vi "Smart_Record_MTIF.vi"() -> ()   [LabVIEW 2019]
uses:
  <vilib>/vision/driver/IMAQdx.llb/IMAQdx Acquisition Mode.ctl
  <vilib>/vision/driver/IMAQdx.llb/IMAQdx Buffer Number Mode.ctl
  <vilib>/vision/driver/NI_Vision_Acquisition_Software.lvlib
  <resource>/objmgr/imaqdx.rc
  <vilib>/vision/NI_Vision_Development_Module.lvlib
panel:
  out "Data Valid":bool
  in  "Centroid Distance Threshold":sgl=5.0
  in  "Initial SD Threshold":sgl=4.0
  in  "SD Threshold Ratio for Stop":sgl=1.2
  in  "SD Threshold Ratio for Start":sgl=1.5
  out "Writing":bool
  in  "Number of Buffered Frames":i32=200
  in  "Smart Record Enable":bool
  out "Actual Frame Rate":dbl=30.03875968992248
  out "Missed Frames":bool
  out "Standard Variation":sgl=5.0659676
  out "Centroid":cluster{"X Centroid":sgl, "Y Centroid":sgl}={"X Centroid"=323.0136, "Y Centroid"=231.01224} {"Y Centroid" format="%.2f"; "X Centroid" format="%.2f"}
  out "Manual ROI":T1={"Global Rectangle"=[216, 122, 424, 344], "Contours"=[{"Contour Type"=0, "ROI Type"=4, "Points"=[216, 122, 424, 344]}]}
  in  "Image Type":T2 items=["Grayscale (U8)", "Grayscale (I16)", "Grayscale (SGL)", "Complex (CSG)", "RGB (U32)", "HSL (U32)", "RGB (U64)", "Grayscale (U16)"]
  in  "Camera Type":enum16{"Basler", "Mako"}(ring)=enum."Mako"
  in  "Folder Path":path=path "C:/Users/Javier Carmona/Documents/LabVIEW Programs/SmartRecord"
  in  "Exposure Time (us)":dbl=10000.0
  out "error out":errorcluster
  in  "Stop":bool
  in  "Byte Order":T3(ring)=enum."little-endian"
  in  "Record?":bool
  in  "File Name (.mtif)":string="test_081519"
  out "Size":cluster{"X":i32, "Y":i32}={"X"=640, "Y"=480}
  out "Actual Camera ROI":T4={"Left"=0, "Top"=0, "Right"=639, "Bottom"=479, "Rotation"=0.0} {"Rotation" format="%.2f"; "Left" scale=0.0..1024.0; "Right" scale=0.0..1024.0}
  in  "Set Camera ROI":T4={"Left"=0, "Top"=0, "Right"=639, "Bottom"=479, "Rotation"=0.0} {"Rotation" min=-90.0 max=90.0 step=1.0 format="%.2f"; "Left" scale=0.0..1024.0; "Right" scale=0.0..1024.0}
  out "Raw Image":T5(plugin-control)
  in  "Frame Rate (fps)":dbl=30.0
  in  "Camera Name":refnum<k21>="cam2" caption="IMAQdx Session"
  in  "error in":errorcluster
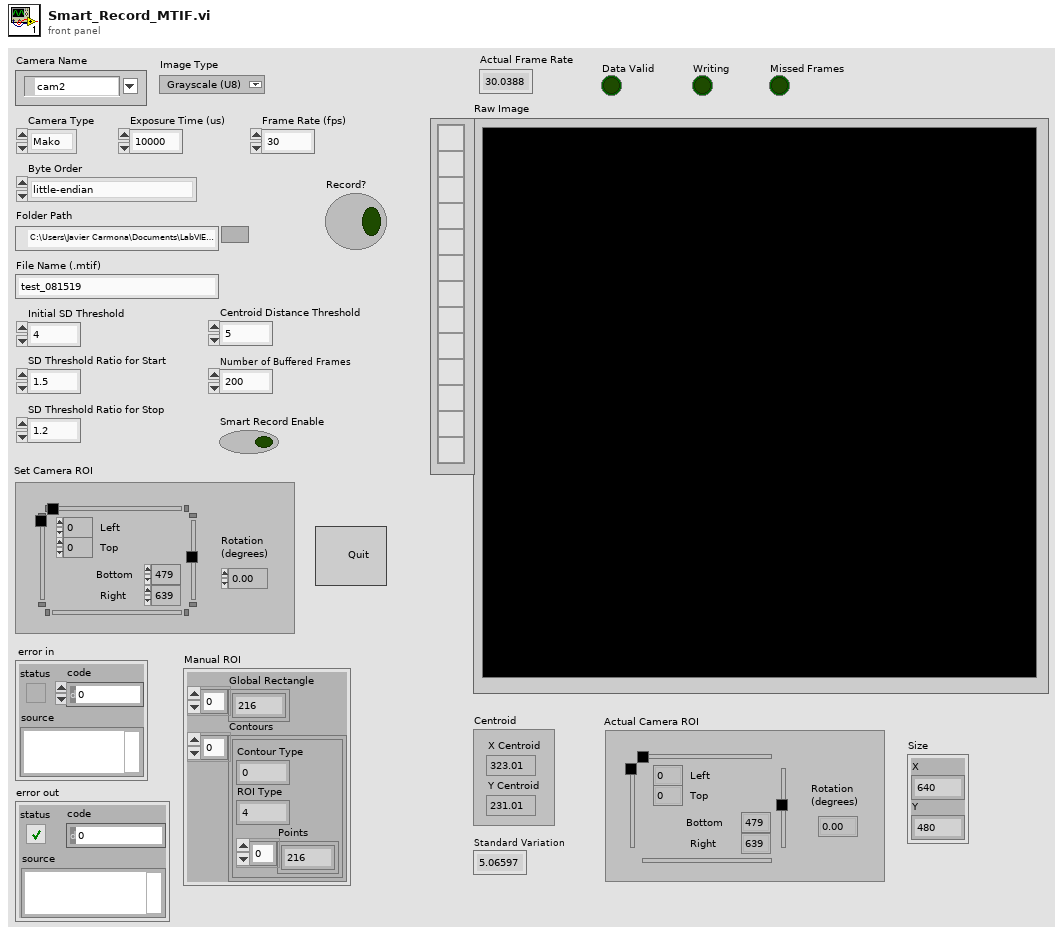
[diagram p1: front panel]
types:
  T1 = cluster{"Global Rectangle":i32[], "Contours":cluster{"Contour Type":u32, "ROI Type":u32, "Points":i32[]}[]}
  T2 = typedef "Image Type" = u32
  T3 = enum16{"big-endian, network order", "native, host order", "little-endian"}
  T4 = typedef "IMAQ Rectangle" = cluster{"Left":i32, "Top":i32, "Right":i32, "Bottom":i32, "Rotation":dbl}
  T5 = typedef "IMAQ Image.ctl" = refnum<image>
  T6 = cluster{"Standard Variation":sgl, "Centroid":cluster{"X Centroid":sgl, "Y Centroid":sgl}}
  T7 = cluster{"ImgDataArray":u8[], "Standard Variation":sgl, "Centroid":cluster{"X Centroid":sgl, "Y Centroid":sgl}}
  T8 = typedef "NI_Vision_Acquisition_Software.lvlib/IMAQdx Acquisition Mode.ctl" = enum32{"One Shot", "Continuous"}
  T9 = typedef "IMAQdx.ctl" = refnum<k21>
  T10 = cluster{"Global Rectangle":i32[], "Contours":cluster{"Contour Type":u32, "Type":u32, "Coordinates":i32[]}[]}
  T11 = cluster{"Mean Value":sgl, "Standard Variation":sgl, "Minimal Value":sgl, "Maximal Value":sgl, "Area (calibrated)":sgl, "Area (pixels)":u32, "%":sgl, "Calibration Valid":bool}
  T12 = typedef "NI_Vision_Acquisition_Software.lvlib/IMAQdx Buffer Number Mode.ctl" = enum32{"Next", "Last", "Buffer Number", "Every", "Last New"}
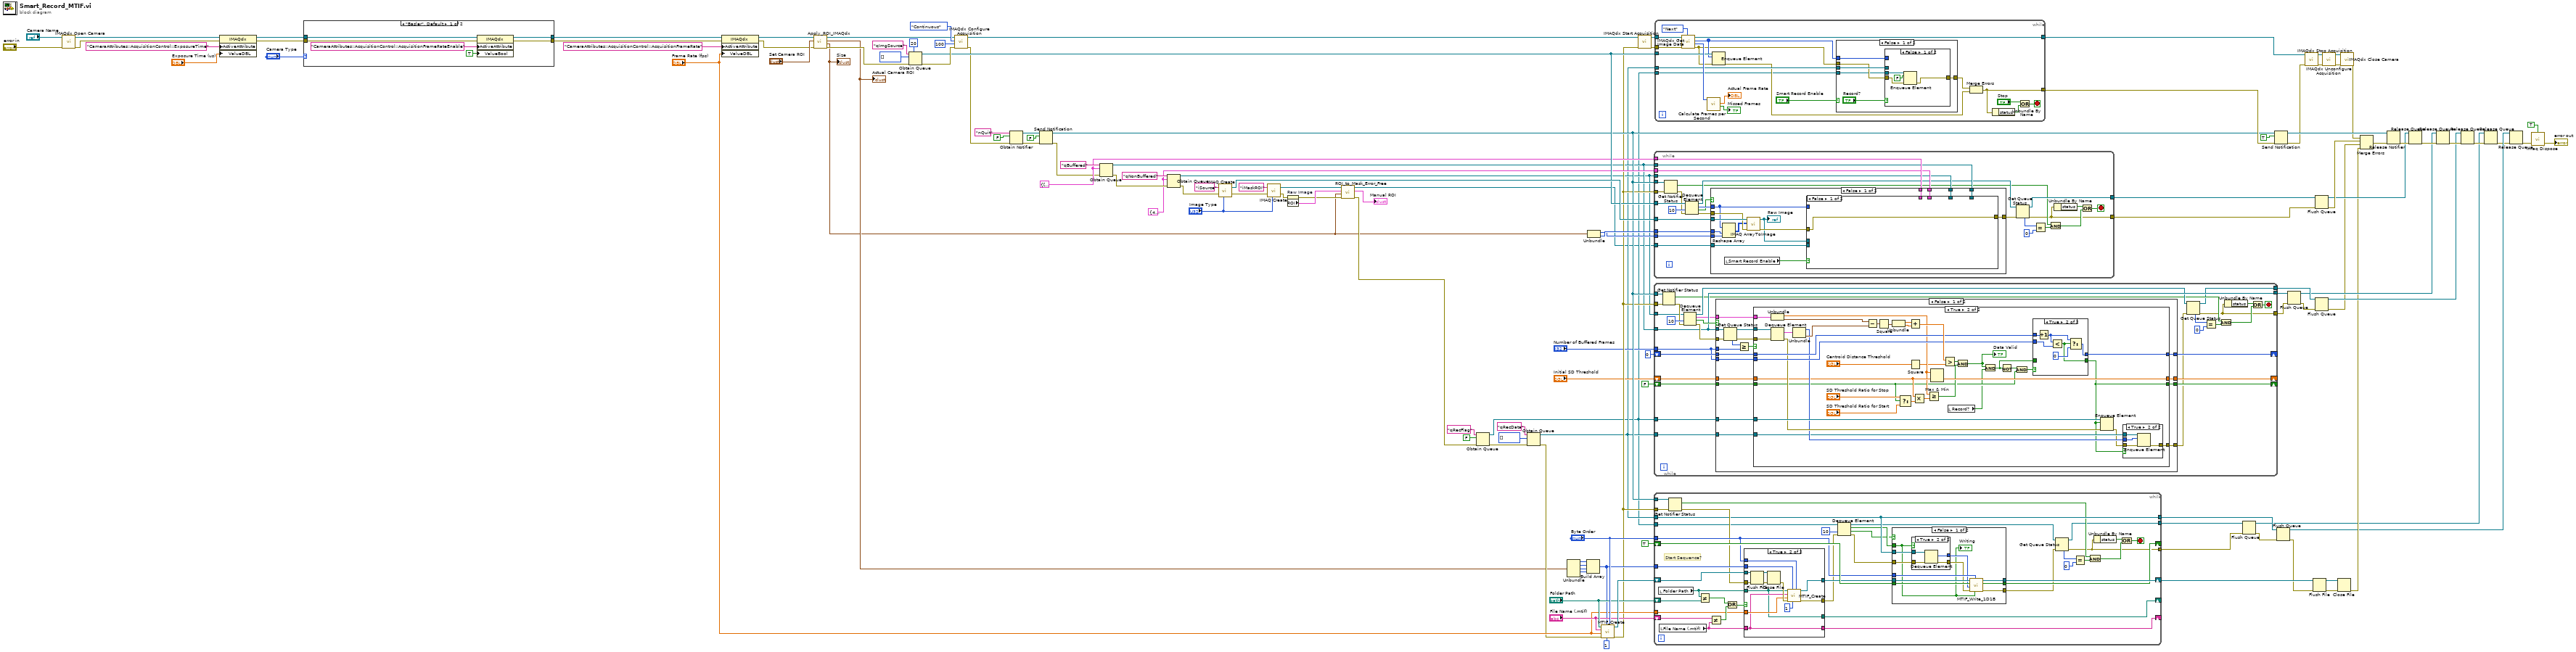
[diagram p0: block diagram]
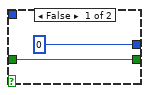
[diagram p4: hidden frame]
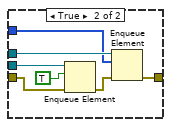
[diagram p6: hidden frame]
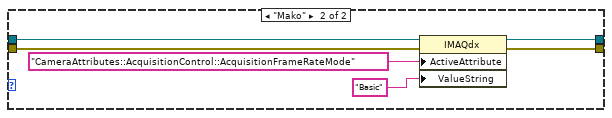
[diagram p8: hidden frame]
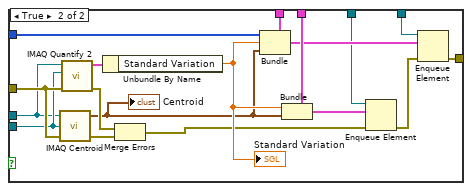
[diagram p9: hidden frame]
diagram:
  w52 = T6 {"Standard Variation"=4836.523, "Centroid"={"X Centroid"=313.66412, "Y Centroid"=260.78278}}
  w53 = T7 {"ImgDataArray"=[], "Standard Variation"=4836.523, "Centroid"={"X Centroid"=313.66412, "Y Centroid"=260.78278}}
  n1 = call <vilib>:"IMAQdx Open Camera.vi"("error in"="error in", "Session In"="Camera Name") -> ("error out"=w82:errorcluster, "Session Out"=w83:T9)  [unwired: 1 in, 7 out]
  n2 = property class="IMAQdx"(reference=w83, error in=w82, "ActiveAttribute"="CameraAttributes::AcquisitionControl::ExposureTime", "ValueDBL"="Exposure Time (us)") -> (reference out=w81:T9, error out=w80:errorcluster)
  n3 = case shown="\"Basler\", Default" "Camera Type" {
    tunnel: w81 -> [w131 w137]
    tunnel: w80 -> [w130 w136]
    tunnel: [w129 w135] -> w79
    tunnel: [w128 w134] -> w78
    frame "Basler", Default {
      n4 = property class="IMAQdx"(reference=w131, error in=w130, "ActiveAttribute"="CameraAttributes::AcquisitionControl::AcquisitionFrameRateEnable", "ValueBool"=TRUE) -> (reference out=w129:T9, error out=w128:errorcluster)
    }
    frame "Mako" {
      n5 = property class="IMAQdx"(reference=w137, error in=w136, "ActiveAttribute"="CameraAttributes::AcquisitionControl::AcquisitionFrameRateMode", "ValueString"="Basic") -> (reference out=w135:T9, error out=w134:errorcluster)
    }
  }
  n6 = property class="IMAQdx"(reference=w79, error in=w78, "ActiveAttribute"="CameraAttributes::AcquisitionControl::AcquisitionFrameRate", "ValueDBL"="Frame Rate (fps)") -> (reference out=w77:T9, error out=w76:errorcluster)
  n7 = call "Apply_ROI_IMAQdx.vi"("error in (no error)"=w76, "ROI"="Set Camera ROI", "Session in"=w77) -> ("error out"=w102:errorcluster, "Size"=w1:cluster{"X":i32, "Y":i32}, "Actual ROI"=w2:T4, "Session out"=w120:T9)  [unwired: 5 in]
  "Actual Camera ROI" <- w2
  "Size" <- w1
  n8 = Obtain Queue(max queue size (-1, unlimited)=20, name (unnamed)="qImgSource", element data type=u8[] [] ("Image Data Array"), error in (no error)=w102) -> (queue out=w62:refnum<queue>, error out=w101:errorcluster)  [unwired: 1 in, 1 out]
  n9 = call <vilib>:"IMAQdx Configure Acquisition.vi"("error in"=w101, "Number of Buffers"=u32 100, "Continuous?"=IMAQdx_Acquisition_Mode."Continuous", "Session In"=w120) -> ("error out"=w50:errorcluster, "Session Out"=w107:T9)  [unwired: 6 in]
  n10 = Obtain Notifier(name (unnamed)="nQuit", notification data type=FALSE ("element"), error in (no error)=w50) -> (notifier out=w97:refnum<notifier>, error out=w96:errorcluster)  [unwired: 1 in, 1 out]
  n11 = Send Notification(notification=FALSE, notifier=w97, error in (no error)=w96) -> (notifier out=w46:refnum<notifier>, error out=w49:errorcluster)
  n12 = Obtain Queue(name (unnamed)="qBuffered", element data type=w53, error in (no error)=w49) -> (queue out=w44:refnum<queue>, error out=w56:errorcluster)  [unwired: 2 in, 1 out]
  n13 = Obtain Queue(name (unnamed)="qNonBuffered", element data type=w52, error in (no error)=w56) -> (queue out=w43:refnum<queue>, error out=w54:errorcluster)  [unwired: 2 in, 1 out]
  n14 = call "IMAQ Create"("Image Name"="iSource", "Image Type"="Image Type", "error in (no error)"=w54) -> ("New Image"=w66:T5, "error out"=w67:errorcluster)  [unwired: 2 in]
  n15 = call "IMAQ Create"("Image Name"="iMaskROI", "Image Type"="Image Type", "error in (no error)"=w67) -> ("New Image"=w8:T5, "error out"=w11:errorcluster)  [unwired: 2 in]
  n16 = property on="Raw Image" class="ImageControl"(error in=w11) -> (error out=w6:errorcluster, "ROI"=w7:T1)  [unwired: 1 in, 1 out]
  n17 = call "ROI_to_Mask_Error_Free.vi"("error in (no error)"=w6, "Image Size"=w1, "ROI in"=w7, "Refnum in"=w8) -> ("error out"=w3:errorcluster, "ROI out"=→"Manual ROI":T10, "Refnum out"=w5:T5)  [unwired: 5 in]
  n18 = Obtain Queue(name (unnamed)="qRecFlag", element data type=FALSE, error in (no error)=w3) -> (queue out=w9:refnum<queue>, error out=w27:errorcluster)  [unwired: 2 in, 1 out]
  n19 = Obtain Queue(name (unnamed)="qRecData", element data type=u8[] [] ("Image Data Array"), error in (no error)=w27) -> (queue out=w10:refnum<queue>, error out=w24:errorcluster)  [unwired: 2 in, 1 out]
  n20 = Unbundle(w2) -> ("Left"=w119:i32, "Top"=w118:i32, "Right"=w117:i32, "Bottom"=w116:i32)  [unwired: 1 out]
  n21 = Build Array(w119, w118, w117, w116) -> (w70:i32[])
  n22 = Unbundle(w1) -> ("X"=w89:i32, "Y"=w90:i32)
  n23 = call "MTIF_Create.vi"("Byte Order"="Byte Order", "Bytes per pixel"=u8 1, "ROI Rectangle"=w70, "error in (no error)"=w24, "Frame Rate (fps)"="Frame Rate (fps)", "File Name (.mtif)"="File Name (.mtif)", "Folder Path"="Folder Path") -> ("error out"=w45:errorcluster, "Byte Stream File out"=w115:refnum<file>)  [unwired: 3 in]
  n24 = call <vilib>:"IMAQdx Start Acquisition.vi"("error in"=w45, "Session In"=w107) -> ("error out"=w63:errorcluster, "Session Out"=w64:T9)  [unwired: 8 in]
  n25 = while {
    tunnel: w46 -> [w164]
    tunnel: w45 -> [w163]
    tunnel: w62 -> [w161]
    tunnel: w90 -> [w158]
    tunnel: w89 -> [w157]
    tunnel: w66 -> [w156]
    tunnel: [w141] -> w88
    tunnel: w5 -> [w154]
    tunnel: w44 -> [w150]
    tunnel: w43 -> [w149]
    tunnel: w53 -> [w152]
    tunnel: w52 -> [w151]
    tunnel: [w138] -> w23
    stop <- w140 stop-if-true
    n26 = Get Notifier Status(notifier=w164, error in (no error)=w163) -> (current notification=w139:bool, error out=w160:errorcluster)  [unwired: 3 out]
    n27 = Dequeue Element(queue=w161, timeout in ms (-1)=10, error in (no error)=w160) -> (queue out=w142:refnum<queue>, element=w159:u8[], timed out?=w153:bool, error out=w155:errorcluster)
    n28 = case shown="False" w153 {
      tunnel: w159 -> [w166 _]
      tunnel: w158 -> [w179 _]
      tunnel: w157 -> [w178 _]
      tunnel: w156 -> [w177 _]
      tunnel: w155 -> [w176 w199]
      tunnel: w154 -> [w173 _]
      tunnel: [w167 w199] -> w143
      tunnel: w152 -> [w172 _]
      tunnel: w151 -> [w170 _]
      tunnel: w150 -> [w169 _]
      tunnel: w149 -> [w168 _]
      frame False {
        n29 = Reshape Array(w166, w179, w178) -> (w171:u8[][])
        n30 = local read "Smart Record Enable"() -> (w165:bool)
        n31 = call "IMAQ ArrayToImage"("error in (no error)"=w176, "Image Pixels (U8)"=w171, "Image"=w177) -> ("error out"=w175:errorcluster, "Image Out"=w174:T5)  [unwired: 7 in]
        "Raw Image" <- w174
        n32 = case shown="False" w165 {
          tunnel: w175 -> [w180 w196]
          tunnel: w174 -> [_ w181]
          tunnel: w173 -> [_ w195]
          tunnel: w172 -> [_ w193]
          tunnel: w170 -> [_ w192]
          tunnel: w169 -> [_ w189]
          tunnel: w168 -> [_ w186]
          tunnel: [w180 w183] -> w167
          tunnel: w166 -> [_ w182]
          frame False {
          }
          frame True {
            n33 = call "IMAQ Centroid"("error in (no error)"=w196, "Image Mask"=w195, "Image"=w181) -> ("error out"=w194:errorcluster, "Centroid"=w190:cluster{"X Centroid":sgl, "Y Centroid":sgl})  [unwired: 1 in]
            "Centroid" <- w190
            n34 = call "IMAQ Quantify 2"("error in (no error)"=w196, "Image Mask"=w195, "Image"=w181) -> ("error out"=w197:errorcluster, "Global Report"=w198:T11)  [unwired: 6 in, 1 out]
            n35 = Unbundle By Name(w198) -> ("Standard Variation"=w191:sgl)
            "Standard Variation" <- w191
            n36 = Merge Errors(w197, w194) -> (w185:errorcluster)
            n37 = Bundle(cluster=w193, "ImgDataArray"=w182, "Standard Variation"=w191, "Centroid"=w190) -> (w188:T7)
            n38 = Bundle(cluster=w192, "Standard Variation"=w191, "Centroid"=w190) -> (w187:T6)
            n39 = Enqueue Element(queue=w186, element=w187, error in (no error)=w185) -> (error out=w184:errorcluster)  [unwired: 1 in, 2 out]
            n40 = Enqueue Element(queue=w189, element=w188, error in (no error)=w184) -> (error out=w183:errorcluster)  [unwired: 1 in, 2 out]
          }
        }
      }
      frame True {
      }
    }
    n41 = Get Queue Status(queue=w142, error in (no error)=w143) -> (queue out=w141:refnum<queue>, error out=w138:errorcluster, # elements in queue=w148:i32)  [unwired: 1 in, 5 out]
    n42 = Equal?(x=w148, y=0) -> (x = y?=w146:bool)
    n43 = And(x=w139, y=w146) -> (x .and. y?=w144:bool)
    n44 = Unbundle By Name(w138) -> ("status"=w145:bool)
    n45 = Or(x=w145, y=w144) -> (x .or. y?=w140:bool)
  }
  n46 = while {
    tunnel: w46 -> [w227]
    tunnel: w45 -> [w225]
    tunnel: w44 -> [w221]
    tunnel: w43 -> [w224]
    tunnel: "Number of Buffered Frames" -> [w215]
    tunnel: [w200] -> w37
    tunnel: [w221] -> w38
    tunnel: [w201] -> w39
    shift-right: [w217] -> _
    shift-left: "Initial SD Threshold" -> [w219]
    shift-right: [w213] -> _
    shift-left: FALSE -> [w220]
    shift-right: [w214] -> _
    shift-left: 0 ("Number of Buffered Frames") -> [w216]
    tunnel: w9 -> [w211]
    tunnel: w10 -> [w212]
    stop <- w204 stop-if-true
    n47 = Get Notifier Status(notifier=w227, error in (no error)=w225) -> (current notification=w205:bool)  [unwired: 4 out]
    n48 = Dequeue Element(queue=w224, timeout in ms (-1)=10, error in (no error)=w225) -> (queue out=w210:refnum<queue>, element=w218:T6, timed out?=w223:bool, error out=w222:errorcluster)
    n49 = case shown="False" w223 {
      tunnel: w222 -> [w244 w304]
      tunnel: [w240 w304] -> w209
      tunnel: w221 -> [w245 _]
      tunnel: w215 -> [w234 _]
      tunnel: w220 -> [w239 w301]
      tunnel: w219 -> [w238 w303]
      tunnel: w218 -> [w237 _]
      tunnel: [w236 w303] -> w217
      tunnel: w216 -> [w233 w302]
      tunnel: w215 -> [w232 _]
      tunnel: [w231 w302] -> w214
      tunnel: [w230 w301] -> w213
      tunnel: w212 -> [w228 _]
      tunnel: w211 -> [w229 _]
      frame False {
        n50 = Get Queue Status(queue=w245, error in (no error)=w244) -> (queue out=w235:refnum<queue>, error out=w241:errorcluster, # elements in queue=w243:i32)  [unwired: 1 in, 5 out]
        n51 = Greater Or Equal?(x=w243, y=w234) -> (x >= y?=w242:bool)
        n52 = case shown="True" w242 {
          tunnel: [w248 w263] -> w240
          tunnel: w241 -> [w248 w282]
          tunnel: w239 -> [w246 w251]
          tunnel: w238 -> [w249 w262]
          tunnel: w237 -> [_ w285]
          tunnel: [w249 w284] -> w236
          tunnel: w235 -> [_ w283]
          tunnel: w233 -> [w247 w271]
          tunnel: w232 -> [_ w270]
          tunnel: [w247 w269] -> w231
          tunnel: [w246 w257] -> w230
          tunnel: w229 -> [_ w268]
          tunnel: w228 -> [_ w265]
          frame False {
          }
          frame True {
            n53 = Dequeue Element(queue=w283, error in (no error)=w282) -> (element=w281:T7, error out=w267:errorcluster)  [unwired: 1 in, 2 out]
            n54 = Unbundle(w285) -> ("Standard Variation"=w261:sgl, "Centroid"=w280:cluster{"X Centroid":sgl, "Y Centroid":sgl})
            n55 = Unbundle(w281) -> ("ImgDataArray"=w266:u8[], "Centroid"=w279:cluster{"X Centroid":sgl, "Y Centroid":sgl})  [unwired: 1 out]
            n56 = Subtract(x=w280, y=w279) -> (x-y=w278:cluster{"X Centroid":sgl, "Y Centroid":sgl})
            n57 = Square(x=w278) -> (x^2=w277:cluster{"X Centroid":sgl, "Y Centroid":sgl})
            n58 = Unbundle(w277) -> ("X Centroid"=w276:sgl, "Y Centroid"=w275:sgl)
            n59 = Select(t="SD Threshold Ratio for Stop", s=w251, f="SD Threshold Ratio for Start") -> (s? t:f=w287:sgl)
            n60 = Add(x=w276, y=w275) -> (x+y=w274:sgl)
            n61 = Square(x="Centroid Distance Threshold") -> (x^2=w255:sgl)
            n62 = Multiply(x=w262, y=w287) -> (x*y=w286:sgl)
            n63 = Greater Or Equal?(x=w261, y=w286) -> (x >= y?=w273:bool)
            n64 = Max & Min(x=w261, y=w262) -> (min(x,y)=w284:sgl)  [unwired: 1 out]
            n65 = Greater?(x=w274, y=w255) -> (0:w272:bool)
            n66 = local read "Record?"() -> (w250:bool)
            n67 = And(x=w272, y=w273) -> (x .and. y?=w256:bool)
            "Data Valid" <- w256
            n68 = And(x=w256, y=w250) -> (x .and. y?=w260:bool)
            n69 = Not(x=w260) -> (.not. x?=w259:bool)
            n70 = And(x=w259, y=w251) -> (x .and. y?=w258:bool)
            n71 = case shown="True" w258 {
              tunnel: w271 -> [_ w300]
              tunnel: [0 w298] -> w269
              tunnel: w270 -> [_ w296]
              tunnel: w260 -> [w293 _]
              tunnel: [w293 w295] -> w257
              frame False {
              }
              frame True {
                n72 = Increment(x=w300) -> (x+1=w297:i32)
                n73 = Less?(x=w297, y=w296) -> (x < y?=w295:bool)
                n74 = Select(t=w297, s=w295, f=0) -> (s? t:f=w298:i32)
              }
            }
            n75 = Enqueue Element(queue=w268, element=w257, error in (no error)=w267) -> (error out=w264:errorcluster)  [unwired: 1 in, 2 out]
            n76 = case shown="True" w257 {
              tunnel: w266 -> [_ w292]
              tunnel: w265 -> [_ w291]
              tunnel: w264 -> [w288 w290]
              tunnel: [w288 w289] -> w263
              frame False {
              }
              frame True {
                n77 = Enqueue Element(queue=w291, element=w292, error in (no error)=w290) -> (error out=w289:errorcluster)  [unwired: 1 in, 2 out]
              }
            }
          }
        }
      }
      frame True {
      }
    }
    n78 = Get Queue Status(queue=w210, error in (no error)=w209) -> (queue out=w200:refnum<queue>, error out=w201:errorcluster, # elements in queue=w208:i32)  [unwired: 1 in, 5 out]
    n79 = Equal?(x=w208, y=0) -> (x = y?=w206:bool)
    n80 = And(x=w205, y=w206) -> (x .and. y?=w202:bool)
    n81 = Unbundle By Name(w201) -> ("status"=w203:bool)
    n82 = Or(x=w203, y=w202) -> (x .or. y?=w204:bool)
  }
  n83 = while {
    tunnel: "Byte Order" -> [w329]
    shift-right: [w340] -> _
    shift-left: TRUE ("Record?") -> [w341]
    shift-right: [w327] -> _
    shift-left: "Folder Path" -> [w339]
    shift-right: [w328] -> _
    shift-left: "File Name (.mtif)" -> [w333]
    tunnel: w70 -> [w330]
    tunnel: "Frame Rate (fps)" -> [w331]
    shift-right: [w342] -> w110
    shift-left: w115 -> [w335]
    tunnel: w46 -> [w325]
    tunnel: w45 -> [w324]
    tunnel: w9 -> [w322]
    tunnel: w10 -> [w318]
    tunnel: [w318] -> w20
    tunnel: [w306] -> w22
    tunnel: [w305] -> w21
    stop <- w307 stop-if-true
    # "Start Sequence?"
    n84 = local read "Folder Path"() -> (w334:path)
    n85 = local read "File Name (.mtif)"() -> (w332:string)
    n86 = Get Notifier Status(notifier=w325, error in (no error)=w324) -> (current notification=w308:bool, error out=w323:errorcluster)  [unwired: 3 out]
    n87 = Not Equal?(x=w334, y=w339) -> (x != y?=w338:bool)
    n88 = Not Equal?(x=w333, y=w332) -> (x != y?=w337:bool)
    n89 = Or(x=w338, y=w337) -> (x .or. y?=w336:bool)
    n90 = case shown="True" w336 {
      tunnel: w335 -> [w365 w378]
      tunnel: w334 -> [w363 w366]
      tunnel: w332 -> [w362 w367]
      tunnel: w323 -> [w364 w377]
      tunnel: [w365 w370] -> w326
      tunnel: [w364 w369] -> w321
      tunnel: w331 -> [_ w373]
      tunnel: w330 -> [_ w371]
      tunnel: w329 -> [_ w368]
      tunnel: [w362 w367] -> w328
      tunnel: [w363 w366] -> w327
      frame False {
      }
      frame True {
        n91 = Flush File(refnum=w378, error in=w377) -> (refnum out=w376:refnum<file>, error out=w375:errorcluster)
        n92 = Close File(refnum=w376, error in=w375) -> (error out=w374:errorcluster)  [unwired: 1 out]
        n93 = call "MTIF_Create.vi"("Byte Order"=w368, "Bytes per pixel"=u8 1, "ROI Rectangle"=w371, "error in (no error)"=w374, "Frame Rate (fps)"=w373, "File Name (.mtif)"=w367, "Folder Path"=w366) -> ("error out"=w369:errorcluster, "Byte Stream File out"=w370:refnum<file>)  [unwired: 3 in]
      }
    }
    n94 = Dequeue Element(queue=w322, timeout in ms (-1)=10, error in (no error)=w321) -> (queue out=w310:refnum<queue>, element=w317:bool, timed out?=w316:bool, error out=w319:errorcluster)
    n95 = case shown="False" w316 {
      tunnel: [w353 w360] -> w342
      tunnel: w341 -> [w352 w361]
      tunnel: [w351 w361] -> w340
      tunnel: w329 -> [w350 _]
      tunnel: w326 -> [w349 w360]
      tunnel: [w348 w359] -> w309
      tunnel: w319 -> [w347 w359]
      tunnel: w318 -> [w346 _]
      tunnel: w317 -> [w343 _]
      frame False {
        n96 = case shown="True" w343 {
          tunnel: w347 -> [w354 w358]
          tunnel: w346 -> [_ w357]
          tunnel: [w354 w356] -> w345
          tunnel: [_ w355] -> w344
          frame False {
          }
          frame True {
            n97 = Dequeue Element(queue=w357, error in (no error)=w358) -> (element=w355:u8[], error out=w356:errorcluster)  [unwired: 1 in, 2 out]
          }
        }
        n98 = call "MTIF_Write_1D1B.vi"("Record?"=w343, "Byte Order"=w350, "error in (no error)"=w345, "Image Data Array"=w344, "Start Sequence? In"=w352, "Byte Stream File In"=w349) -> ("error out"=w348:errorcluster, "Start Sequence? Out"=w351:bool, "Byte Stream File Out"=w353:refnum<file>)  [unwired: 3 in]
        "Writing" <- w343
      }
      frame True {
      }
    }
    n99 = Get Queue Status(queue=w310, error in (no error)=w309) -> (queue out=w306:refnum<queue>, error out=w305:errorcluster, # elements in queue=w315:i32)  [unwired: 1 in, 5 out]
    n100 = Equal?(x=w315, y=0) -> (x = y?=w313:bool)
    n101 = And(x=w308, y=w313) -> (x .and. y?=w311:bool)
    n102 = Unbundle By Name(w305) -> ("status"=w312:bool)
    n103 = Or(x=w312, y=w311) -> (x .or. y?=w307:bool)
  }
  n104 = while {
    tunnel: w64 -> [w396]
    tunnel: w63 -> [w395]
    tunnel: [w392] -> w60
    tunnel: w62 -> [w389]
    tunnel: [w383] -> w59
    tunnel: w10 -> [w386]
    tunnel: w9 -> [w379]
    stop <- w391 stop-if-true
    n105 = call <vilib>:"IMAQdx Get Image Data.vi"("Buffer Number Mode (Next)"=IMAQdx_Buffer_Number_Mode."Next", "error in"=w395, "Session In"=w396) -> ("error out"=w384:errorcluster, "Buffer Number Out"=w393:u32, "Image Data Array"=w385:u8[], "Session Out"=w392:T9)  [unwired: 5 in]
    n106 = call <vilib>:"Calculate Frames per Second.vi"("Buffer Number"=w393) -> ("Missed Frames"=→"Missed Frames":bool, "Processed Frames/s"=→"Actual Frame Rate":dbl)  [unwired: 8 in, 1 out]
    n107 = Enqueue Element(queue=w389, element=w385, error in (no error)=w384) -> (error out=w382:errorcluster)  [unwired: 1 in, 2 out]
    n108 = case shown="False" "Smart Record Enable" {
      tunnel: w386 -> [w403 _]
      tunnel: w384 -> [w402 w415]
      tunnel: w385 -> [w401 _]
      tunnel: [w400 w415] -> w381
      tunnel: w379 -> [w398 _]
      frame False {
        n109 = case shown="False" "Record?" {
          tunnel: w403 -> [_ w414]
          tunnel: w402 -> [w406 w410]
          tunnel: w401 -> [_ w413]
          tunnel: [w404 w412] -> w400
          tunnel: w398 -> [w407 w411]
          frame False {
            n110 = Enqueue Element(queue=w407, element=FALSE, error in (no error)=w406) -> (error out=w404:errorcluster)  [unwired: 1 in, 2 out]
          }
          frame True {
            n111 = Enqueue Element(queue=w411, element=TRUE, error in (no error)=w410) -> (error out=w408:errorcluster)  [unwired: 1 in, 2 out]
            n112 = Enqueue Element(queue=w414, element=w413, error in (no error)=w408) -> (error out=w412:errorcluster)  [unwired: 1 in, 2 out]
          }
        }
      }
      frame True {
      }
    }
    n113 = Merge Errors(w381, w382) -> (w383:errorcluster)
    n114 = Unbundle By Name(w383) -> ("status"=w390:bool)
    n115 = Or(x="Stop", y=w390) -> (x .or. y?=w391:bool)
  }
  n116 = Flush Queue(queue=w22, error in (no error)=w21) -> (queue out=w16:refnum<queue>, error out=w19:errorcluster)  [unwired: 1 out]
  n117 = Send Notification(notification=TRUE, notifier=w46, error in (no error)=w59) -> (notifier out=w93:refnum<notifier>, error out=w58:errorcluster)
  n118 = Flush Queue(queue=w20, error in (no error)=w19) -> (queue out=w15:refnum<queue>, error out=w18:errorcluster)  [unwired: 1 out]
  n119 = Flush Queue(queue=w38, error in (no error)=w39) -> (queue out=w34:refnum<queue>, error out=w36:errorcluster)  [unwired: 1 out]
  n120 = call <vilib>:"IMAQdx Stop Acquisition.vi"("error in"=w58, "Session In"=w60) -> ("error out"=w113:errorcluster, "Session Out"=w114:T9)  [unwired: 8 in]
  n121 = Flush File(refnum=w110, error in=w18) -> (refnum out=w109:refnum<file>, error out=w108:errorcluster)
  n122 = Flush Queue(queue=w88, error in (no error)=w23) -> (queue out=w47:refnum<queue>, error out=w48:errorcluster)  [unwired: 1 out]
  n123 = Flush Queue(queue=w37, error in (no error)=w36) -> (queue out=w35:refnum<queue>, error out=w33:errorcluster)  [unwired: 1 out]
  n124 = call <vilib>:"IMAQdx Unconfigure Acquisition.vi"("error in"=w113, "Session In"=w114) -> ("error out"=w112:errorcluster, "Session Out"=w111:T9)  [unwired: 8 in]
  n125 = Close File(refnum=w109, error in=w108) -> (error out=w32:errorcluster)  [unwired: 1 out]
  n126 = call <vilib>:"IMAQdx Close Camera.vi"("error in"=w112, "Session In"=w111) -> ("error out"=w61:errorcluster)  [unwired: 9 out]
  n127 = Merge Errors(w61, w48, w33, w32) -> (w94:errorcluster)
  n128 = Release Notifier(notifier=w93, error in (no error)=w94) -> (error out=w51:errorcluster)  [unwired: 1 in, 2 out]
  n129 = Release Queue(queue=w47, error in (no error)=w51) -> (error out=w41:errorcluster)  [unwired: 1 in, 2 out]
  n130 = Release Queue(queue=w34, error in (no error)=w41) -> (error out=w40:errorcluster)  [unwired: 1 in, 2 out]
  n131 = Release Queue(queue=w35, error in (no error)=w40) -> (error out=w17:errorcluster)  [unwired: 1 in, 2 out]
  n132 = Release Queue(queue=w16, error in (no error)=w17) -> (error out=w14:errorcluster)  [unwired: 1 in, 2 out]
  n133 = Release Queue(queue=w15, error in (no error)=w14) -> (error out=w13:errorcluster)  [unwired: 1 in, 2 out]
  n134 = call "Imaq Dispose"("All Images? (No)"=TRUE, "error in (no error)"=w13) -> ("error out"=→"error out":errorcluster)  [unwired: 1 in, 3 out]
